vi "SRXGetAbsoluteOffset.vi"(1 "QuadPosition":i32, 2 "AbsolutePosition (No Overflow)":i32) -> (0 "Offset":i32)   [LabVIEW 2018]
uses:
  14c67783-24ae-4a51-9213-2a54079da666.vi
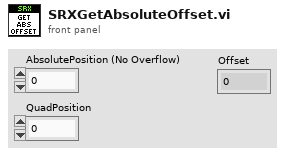
[diagram p1: front panel]
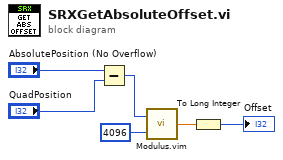
[diagram p0: block diagram]
diagram:
  n1 = Subtract(x="AbsolutePosition (No Overflow)", y="QuadPosition") -> (x-y=w4:i32)
  n2 = call "Modulus.vim"("y"=4096 ("x-y"), "x"=w4) -> ("x%y"=w2:dbl)
  n3 = To Long Integer(number=w2) -> (32bit integer=→"Offset":i32)
